vi "REPORT_OKNOK_prepare_header_for_pdf.vi"(11 "REPORT_OKNOK_all_info":T1) -> (3 "report_header":string[][](array[string]))   [LabVIEW 2019]
uses:
  typedef/REPORT_OKNOK_all_info.ctl
  _misc/AULocalize/SubVIs/Get Localized Phrase Compact Interface 1D.vi
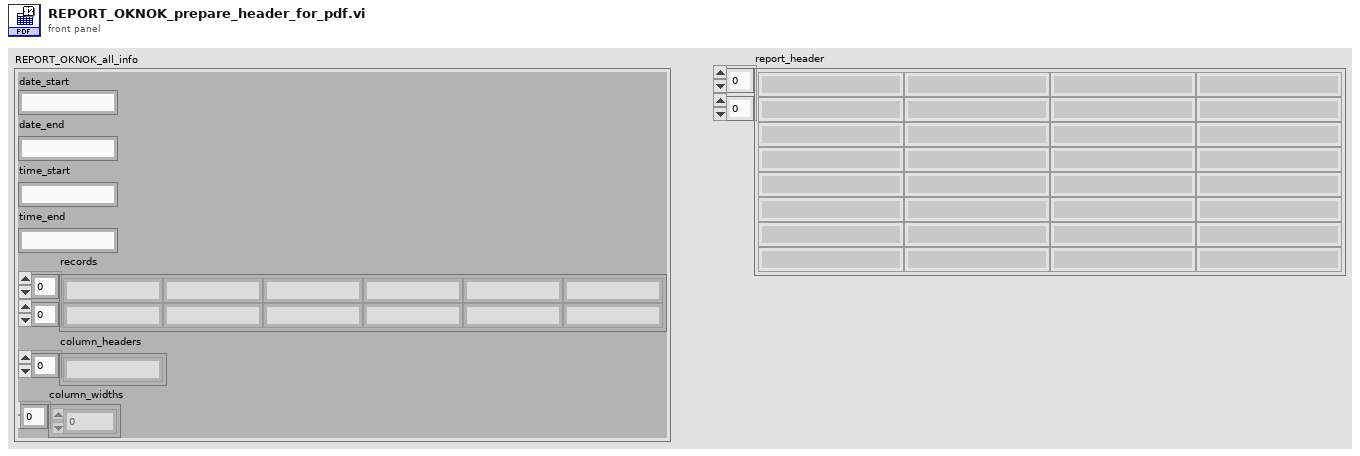
[diagram p1: front panel]
types:
  T1 = typedef "REPORT_OKNOK_all_info.ctl" = cluster{"date_start":string, "date_end":string, "time_start":string, "time_end":string, "records":string[][], "column_headers":string[], "column_widths":i16[]}
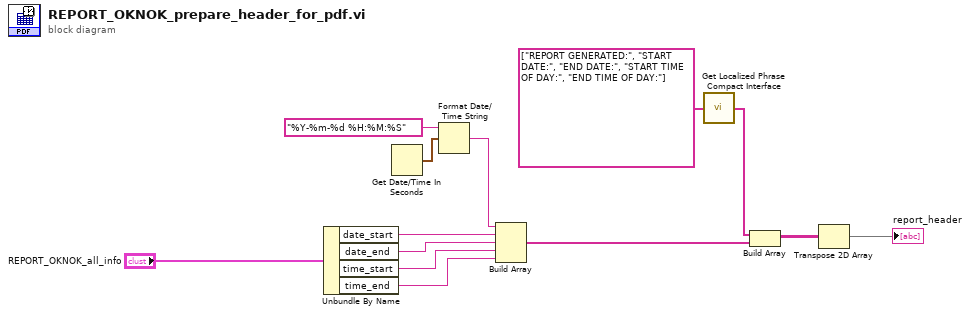
[diagram p0: block diagram]
diagram:
  n1 = Unbundle By Name("REPORT_OKNOK_all_info") -> ("date_start"=w6:string, "date_end"=w5:string, "time_start"=w4:string, "time_end"=w3:string)
  n2 = Get Date/Time In Seconds() -> (seconds since 1Jan1904=w12:timestamp)
  n3 = Format Date/Time String(time format string (%c)="%Y-%m-%d %H:%M:%S", seconds (now)=w12) -> (date/time string=w7:string)  [unwired: 1 in]
  n4 = Build Array(w7, w6, w5, w4, w3) -> (w8:string[])
  n5 = call-poly "Get Localized Phrase Compact Interface.vi"("Key"=string[] ["REPORT GENERATED:", "START DATE:", "END DATE:", "START TIME OF DAY:", "END TIME OF DAY:"]) -> ("Translated Phrase"=w1:string[])
  n6 = Build Array(w1, w8) -> (w10:string[][])
  n7 = Transpose 2D Array(2D array=w10) -> (transposed array=→"report_header":string[][])
